vi "Set Relays (Batch).vi"(0 "connection ID":refnum<k16>, 1 "address":u32, 2 "port":u16, 5 "Mask":bool[](array[boolean])=[TRUE, TRUE, TRUE, TRUE, TRUE, TRUE, TRUE, TRUE, TRUE, TRUE, TRUE, TRUE, TRUE, TRUE, TRUE, TRUE], 7 "Relay State":T1 items=["LOW", "HIGH"], 9 "timeout ms (1000)":i32=1000, 11 "error in (no error)":errorcluster) -> (4 "connection ID out":refnum<k16>, 6 "received data":string, 15 "error out":errorcluster)   [LabVIEW 2016, in "instr.lvlib"]
doc: "Sets all relays to a given state. Batch operation."
uses:
  instr.lvlib
  IO State.ctl
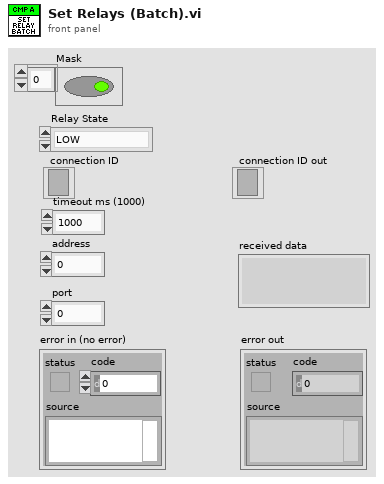
[diagram p1: front panel]
types:
  T1 = typedef "instr.lvlib/IO State.ctl" = u16
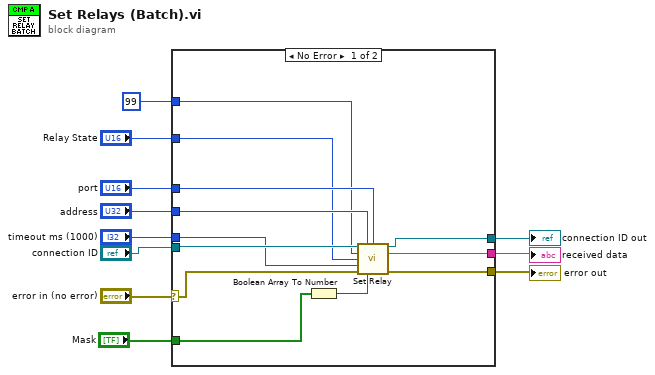
[diagram p0: block diagram]
diagram:
  n1 = case shown="No Error" "error in (no error)" {
    selector: "error in (no error)" -> [w21 w25]
    tunnel: [w23 w25] -> w11
    tunnel: "timeout ms (1000)" -> [w15 _]
    tunnel: "connection ID" -> [w20 w24]
    tunnel: [w22 w24] -> w7
    tunnel: u16 99 ("Relay Number") -> [w17 _]
    tunnel: "Relay State" -> [w16 _]
    tunnel: "address" -> [w18 _]
    tunnel: "port" -> [w19 _]
    tunnel: [w14 _] -> w2
    tunnel: "Mask" -> [w12 _]
    frame No Error {
      n2 = Boolean Array To Number(Boolean array=w12) -> (number=w13:u32)
      n3 = call "Set Relay.vi"("connection ID"=w20, "address"=w18, "port"=w19, "Relay Number"=w17, "Relay State"=w16, "timeout ms (1000)"=w15, "error in (no error)"=w21, "mask"=w13) -> ("connection ID out"=w22:refnum<k16>, "received data"=w14:string, "error out"=w23:errorcluster)  [unwired: 5 in]
    }
    frame Error {
    }
  }
  "error out" <- w11
  "received data" <- w2
  "connection ID out" <- w7
